vi "Switch Cal Standard.vi"(0 "Manual Cal Standard in":refnum<class "Cal Standard.lvclass">, 5 "Standard Type":T1, 7 "Path Name":string, 11 "error in (no error)":errorcluster) -> (4 "Manual Cal Standard out":refnum<class "Cal Standard.lvclass">, 15 "error out":errorcluster)   [LabVIEW 2023, in "Manual Cal Standard.lvlib" / "Cal Standard.lvclass"]
uses:
  Cal Standard.lvclass
  Instruments/Cal Standard/Type Definitions/Standard Type.ctl
  Common/RFCalAndFixtureCharact.Common.lvlib
  Instruments/RFFixtureCharact.Instruments.lvlib
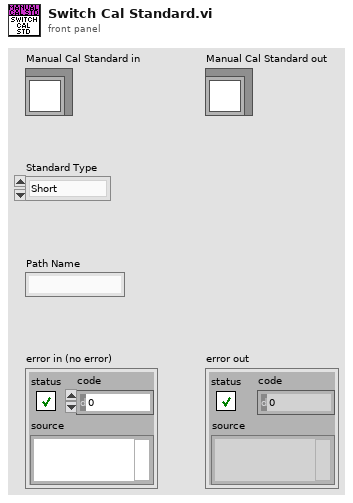
[diagram p1: front panel]
types:
  T1 = typedef "RFFixtureCharact.Instruments.lvlib/Standard Type.ctl" = enum16{"Short", "Open", "Load"}
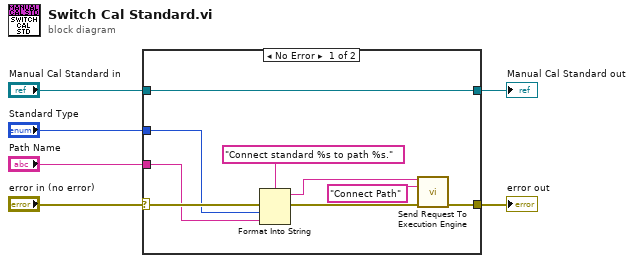
[diagram p0: block diagram]
diagram:
  n1 = case shown="No Error" "error in (no error)" {
    selector: "error in (no error)" -> [w12 w17]
    tunnel: [w15 w17] -> w3
    tunnel: [w11 w16] -> w5
    tunnel: "Manual Cal Standard in" -> [w11 w16]
    tunnel: "Standard Type" -> [w10 _]
    tunnel: "Path Name" -> [w9 _]
    frame No Error {
      n2 = Format Into String(format string="Connect standard %s to path %s.", error in=w12, w10, w9) -> (resulting string=w8:string, error out=w14:errorcluster)  [unwired: 1 in]
      n3 = call "Send Request To Execution Engine.vi"("Request Message"=w8, "Request Header"="Connect Path", "error in (no error)"=w14) -> ("error out"=w15:errorcluster)  [unwired: 11 in, 1 out]
    }
    frame Error {
    }
  }
  "error out" <- w3
  "Manual Cal Standard out" <- w5
